vi "Construct.vi"(1 "Color":u32(colorbox), 2 "Radius":dbl) -> (0 "Draw Component out":refnum<class "DrawComponent.lvclass">)   [LabVIEW 2022 SP3, in "DrawComponent.lvclass"]
uses:
  DrawComponent.lvclass
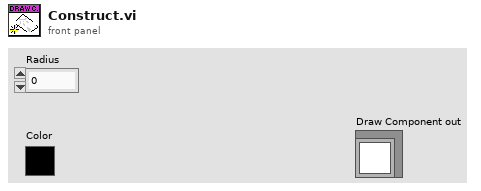
[diagram p1: front panel]
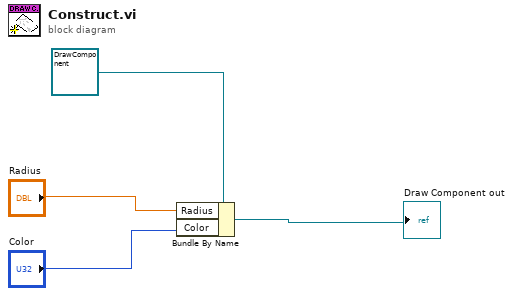
[diagram p0: block diagram]
diagram:
  n1 = Bundle By Name(cluster=refnum<class "DrawComponent.lvclass"> refnum ("DrawComponent.lvclass"), "Radius"="Radius", "Color"="Color") -> (→"Draw Component out":refnum<class "DrawComponent.lvclass">)
